vi "Try1_TCP.vi"() -> ()   [LabVIEW 2024]
panel:
  out "data out":string
  in  "bytes to read":i32
  in  "stop":bool
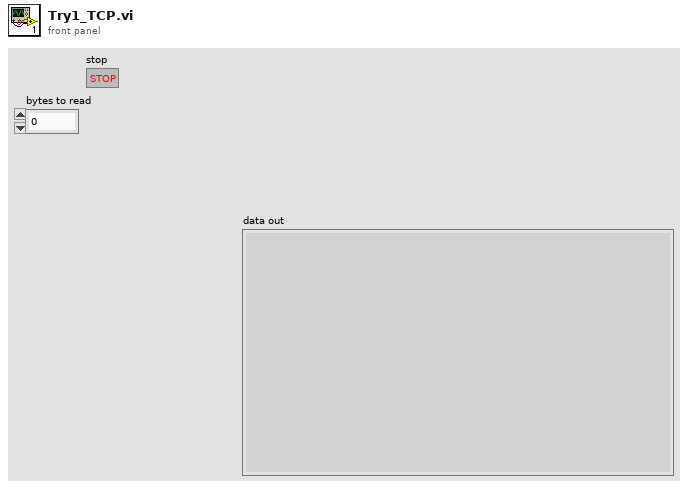
[diagram p1: front panel]
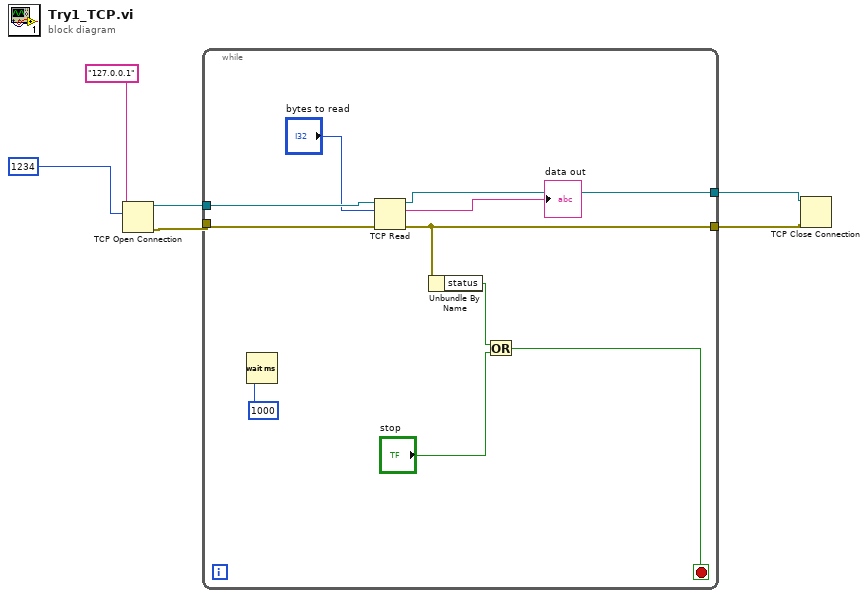
[diagram p0: block diagram]
diagram:
  n1 = TCP Open Connection(address="127.0.0.1", remote port or service name=u16 1234 ("puerto")) -> (connection ID=w4:refnum<k5>, error out=w3:errorcluster)  [unwired: 3 in]
  n2 = while {
    tunnel: w4 -> [w16]
    tunnel: w3 -> [w15]
    tunnel: [w10] -> w2
    tunnel: [w14] -> w1
    stop <- w12 stop-if-true
    n3 = Wait (ms)(milliseconds to wait=u32 1000 ("millisecond timer value")) -> ()  [unwired: 1 out]
    n4 = TCP Read(connection ID=w16, bytes to read="bytes to read", error in (no error)=w15) -> (connection ID out=w14:refnum<k5>, data out=→"data out":string, error out=w10:errorcluster)  [unwired: 2 in]
    n5 = Unbundle By Name(w10) -> ("status"=w11:bool)
    n6 = Or(x=w11, y="stop") -> (x .or. y?=w12:bool)
  }
  n7 = TCP Close Connection(connection ID=w1, error in (no error)=w2) -> ()  [unwired: 1 in, 2 out]
